vi "readFromXML.vi"(8 "error in (no error)":errorcluster, 10 "XML in":string, 11 "MccRotMove in":refnum<class "MccRotMove.lvclass">) -> (0 "error out":errorcluster, 3 "MccRotMove out":refnum<class "MccRotMove.lvclass">)   [LabVIEW 2022 SP3, in "TCSDataDefinitions.lvlib" / "TCSMountControlCommand.lvlib" / "CommandsForRotatorAxis.lvlib" / "MccRotMove.lvclass"]
uses:
  MccRotMove.lvclass
  <userlib>/Common/UnitsAndXML/FlattenItemWithUnitToXML/FlattenPlaneAngleToXML/PlaneAngleUnit.ctl
  MccRotMove.lvclass/MccRotMove.ctl
  CommandsForRotatorAxis.lvclass
  <userlib>/Common/UnitsAndXML/UnitsAndXML.lvlib
  <userlib>/Common/XML/XMLParser/XMLParser.lvclass
panel:
  out "rotAngle":dbl[unit]
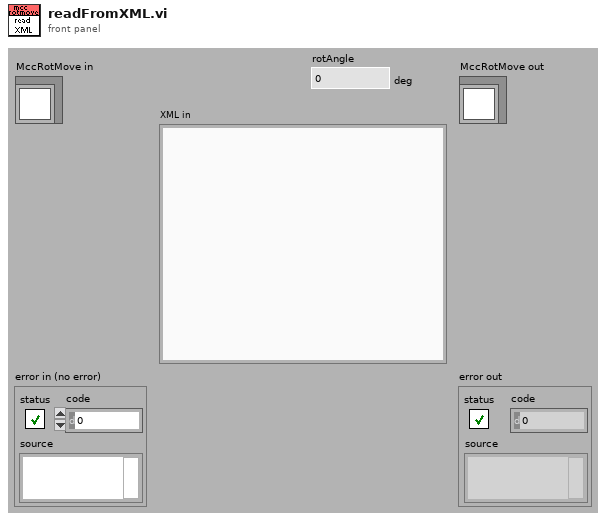
[diagram p1: front panel]
types:
  T1 = typedef "UnitsAndXML.lvlib/PlaneAngleUnit.ctl" = enum16{"rad", "deg", "'", "\""}
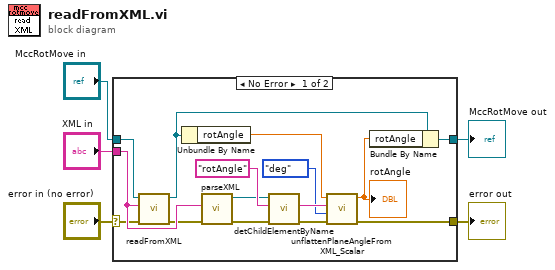
[diagram p0: block diagram]
diagram:
  n1 = case shown="No Error" "error in (no error)" {
    selector: "error in (no error)" -> [w15 w22]
    tunnel: [w7 w22] -> w4
    tunnel: [w10 w21] -> w2
    tunnel: "MccRotMove in" -> [w20 w21]
    tunnel: "XML in" -> [w18 _]
    frame No Error {
      n2 = call-parent "readFromXML.vi"("error in (no error)"=w15, "XML in"=w18, "CommandsForRotatorAxis in"=w20) -> ("error out"=w17:errorcluster, "CommandsForRotatorAxis out"=w14:refnum<class "MccRotMove.lvclass">)  [unwired: 7 out]
      n3 = Unbundle By Name(w14) -> ("rotAngle"=w12:dbl[unit])
      n4 = call <userlib>:"parseXML.vi"("error in (no error)"=w17, "XMLString in"=w18) -> ("error out"=w16:errorcluster, "Element out"=w6:refnum<class "XMLParser.lvclass">)  [unwired: 8 in]
      n5 = call <userlib>:"detChildElementByName.vi"("error in (no error)"=w16, "childName"="rotAngle" ("ChildName"), "Element in"=w6) -> ("error out"=w8:errorcluster, "childXML"=w13:string)  [unwired: 5 in, 2 out]
      n6 = call <userlib>:"unflattenPlaneAngleFromXML_Scalar.vi"("error in (no error)"=w8, "planeAngleUnitInXML"=PlaneAngleUnit."deg", "xmlString"=w13, "planeAngleForType"=w12) -> ("error out"=w7:errorcluster, "planeAngle"=w11:dbl[unit])  [unwired: 6 in]
      "rotAngle" <- w11
      n7 = Bundle By Name(cluster=w14, "rotAngle"=w11) -> (w10:refnum<class "MccRotMove.lvclass">)
    }
    frame Error {
    }
  }
  "error out" <- w4
  "MccRotMove out" <- w2
